vi "Modify IO Pin Enable Array.vi"(7 "VI to Code Relative Path":string="IONode\\SPIEngineSOM.vi", 8 "Error In":errorcluster, 10 "Enable":bool[](array[boolean])=[TRUE, FALSE, TRUE], 11 "Source Root Path":path=path "C:/Users/kvemishe/Downloads/TestScript") -> (0 "Error Out":errorcluster, 1 "Found Object?":bool, 3 "Source Root Path Out":path=path "C:/Users/kvemishe/Downloads/IONode/DLULayer/Dequeue Cmds From Nodes.vi")   [LabVIEW 2014]
doc: "This VI scripts the deque commands VI for the IO Node Engine"
uses:
  <vilib>/Utility/traverseref.llb/TRef TravTarget.ctl
  <vilib>/Utility/traverseref.llb/VI Scripting - Traverse.lvlib
panel:
  out "NumCasesFound":i32
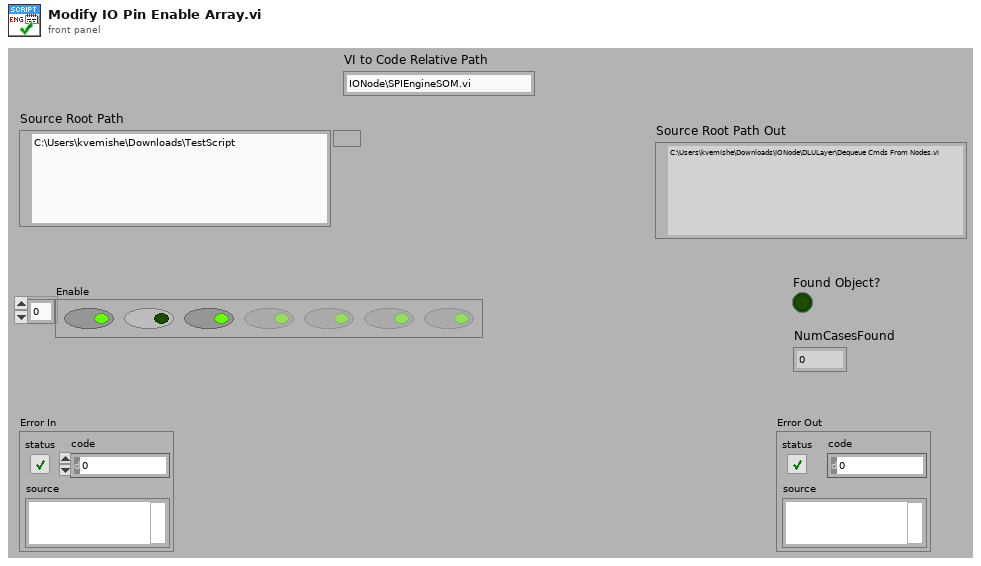
[diagram p1: front panel]
types:
  T1 = typedef "TRef TravTarget.ctl" = enum16{"FP", "BD", "Other"}
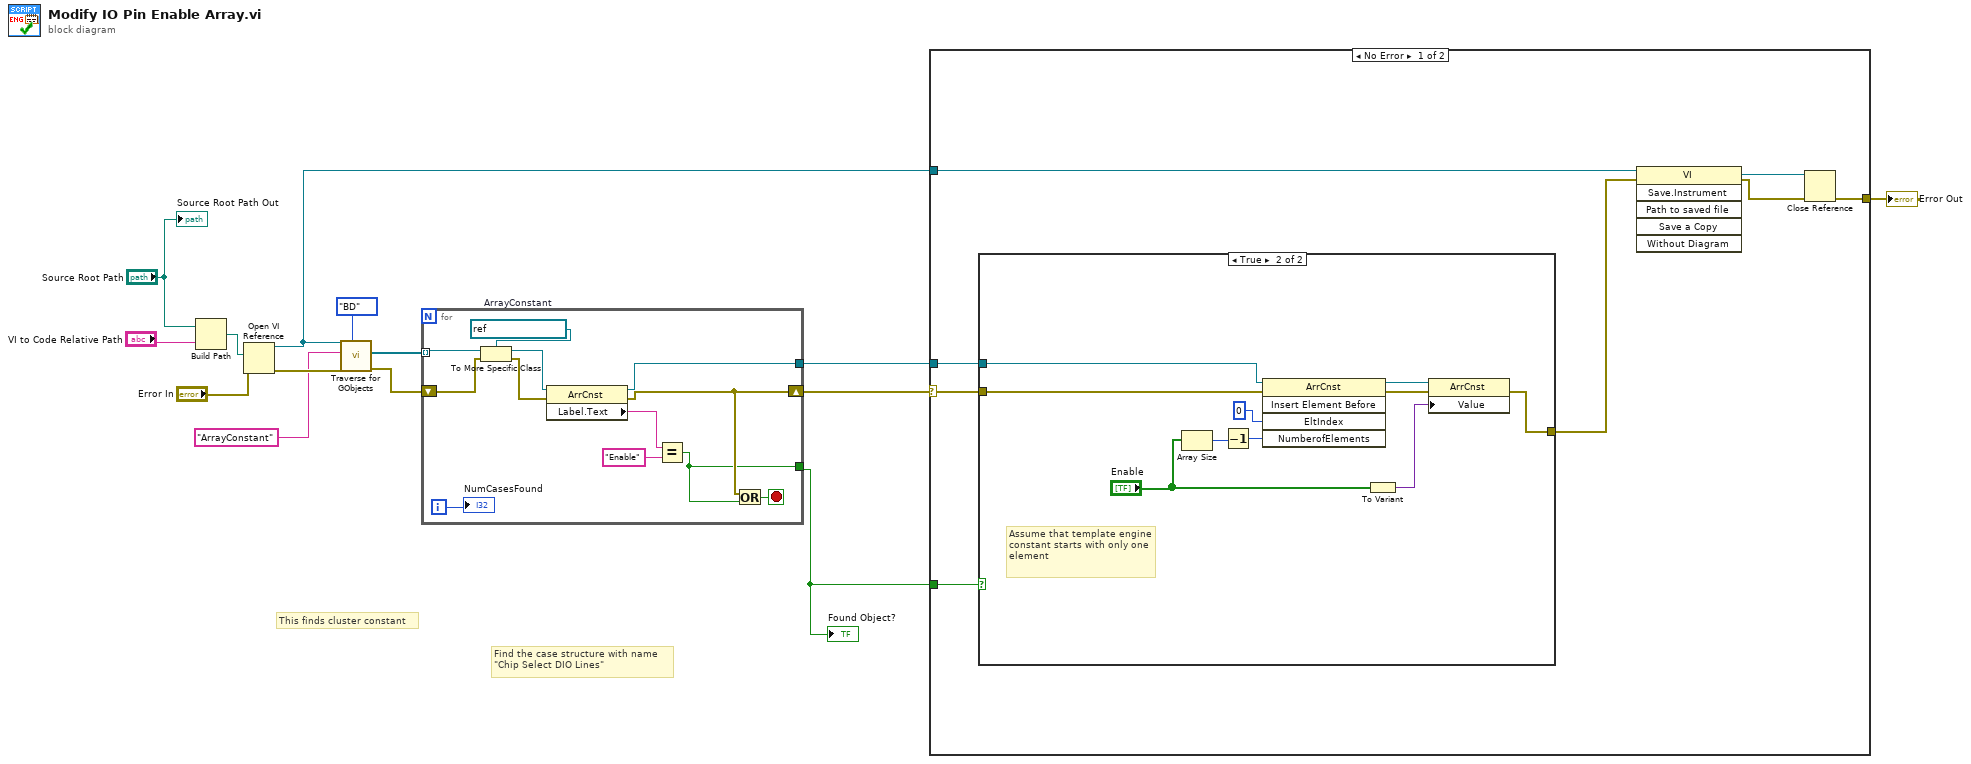
[diagram p0: block diagram]
diagram:
  # "Find the case structure with name\n\"Chip Select DIO Lines\""
  # "This finds cluster constant"
  n1 = Build Path(base path="Source Root Path", name or relative path="VI to Code Relative Path") -> (appended path=w4:path)
  n2 = Open VI Reference(vi path=w4, error in (no error)="Error In") -> (vi reference=w1:refnum<vi>, error out=w13:errorcluster)  [unwired: 4 in]
  n3 = call <vilib>:"Traverse for GObjects.vi"("Traverse Target"=TRef_TravTarget."BD", "error in (no error)"=w13, "Class Name"="ArrayConstant", "VI Refnum"=w1) -> ("error out"=w10:errorcluster, "References"=w11:refnum<vi>[])  [unwired: 4 in, 2 out]
  n4 = for {
    tunnel: w11 -> [w26] mode=indexing
    shift-right: [w18] -> w8
    shift-left: w10 -> [w24]
    tunnel: [w17] -> w7
    tunnel: [w16] -> w9
    i -> [w15]
    stop <- w19 stop-if-true
    w25 = refnum<vi> refnum  # ArrayConstant
    n5 = To More Specific Class(target class=w25, reference=w26, error in=w24) -> (specific class reference=w23:refnum<vi>, error out=w22:errorcluster)
    n6 = property class="ArrCnst"(reference=w23, error in=w22) -> (reference out=w16:refnum<vi>, error out=w18:errorcluster, "Label.Text"=w21:string)
    n7 = Equal?(x=w21, y="Enable") -> (x = y?=w17:bool)
    n8 = Or(x=w18, y=w17) -> (x .or. y?=w19:bool)
    "NumCasesFound" <- w15
  }
  "Found Object?" <- w7
  n9 = case shown="No Error" w8 {
    selector: w8 -> [w32 w46]
    tunnel: w9 -> [w34 _]
    tunnel: w7 -> [w33 _]
    tunnel: w1 -> [w28 _]
    tunnel: [w27 w46] -> w5
    frame No Error {
      n10 = case shown="True" w33 {
        tunnel: w34 -> [_ w39]
        tunnel: w32 -> [w35 w42]
        tunnel: [w35 w45] -> w29
        frame False {
        }
        frame True {
          # "Assume that template engine constant starts with only one element"
          n11 = Array Size(array="Enable") -> (size(s)=w44:i32)
          n12 = Decrement(x=w44) -> (x-1=w43:i32)
          n13 = invoke class="ArrCnst" method="Insert Element Before"(reference=w39, error in=w42, "EltIndex"=0 ("Element Index"), "NumberofElements"=w43) -> (reference out=w40:refnum<vi>, error out=w41:errorcluster)  [unwired: 1 in, 3 out]
          n14 = To Variant(anything="Enable") -> (Variant=w36:variant)
          n15 = property class="ArrCnst"(reference=w40, error in=w41, "Value"=w36) -> (error out=w45:errorcluster)  [unwired: 1 out]
        }
      }
      n16 = invoke class="VI" method="Save.Instrument"(reference=w28, error in=w29) -> (reference out=w31:refnum<vi>, error out=w30:errorcluster)  [unwired: 4 in, 4 out]
      n17 = Close Reference(reference=w31, error in (no error)=w30) -> (error out=w27:errorcluster)
    }
    frame Error {
    }
  }
  "Error Out" <- w5
  "Source Root Path Out" <- "Source Root Path"
